vi "Actor Core.vi"(8 "error in":errorcluster, 11 "FlexUIActorTemplate in":refnum<class "FlexUIActorTemplate.lvclass">) -> (0 "error out":errorcluster, 3 "Actor out":refnum<class "Actor.lvclass">)   [LabVIEW 2016, in "FlexUIActorTemplate.lvlib" / "FlexUIActorTemplate.lvclass"]
doc: "(<B>Filename</B>: Actor Framework.lvlib:Actor.lvclass:Actor Core.vi)\n\nReceives messages to the actor, reacts to them, and initiates any error handling that may shut the actor down.\n\nDescendant classes may override this VI to append parallel tasks for the actor to complete while it handles messages. Overrides use the Call Parent Method node."
uses:
  FlexUIActorTemplate.lvclass
  <vilib>/ActorFramework/Actor/Actor.lvclass
  Flex UI Dialog (Actor) Messages/Publish UI Closed Msg/Publish UI Closed Msg.lvclass
  <vilib>/ActorFramework/Stop Msg/Stop Msg.lvclass
  Flex UI Dialog (Actor)/Flex Dialog (Actor).lvclass
  E:/LabVIEW/VI Packages/Flex UI (Actor)/Flex UI Dialog (Actor)/Flex Dialog (Actor).lvclass
  E:/LabVIEW/VI Packages/Flex UI (Actor)/Flex UI (Actor)/Flex UI (Actor).lvclass
  C:/Program Files (x86)/National Instruments/LabVIEW 2016/vi.lib/East West Architects/Parent Actor Template/_Parent Actor Template.lvclass
  C:/Program Files (x86)/National Instruments/LabVIEW 2016/vi.lib/ActorFramework/Actor/Actor.lvclass
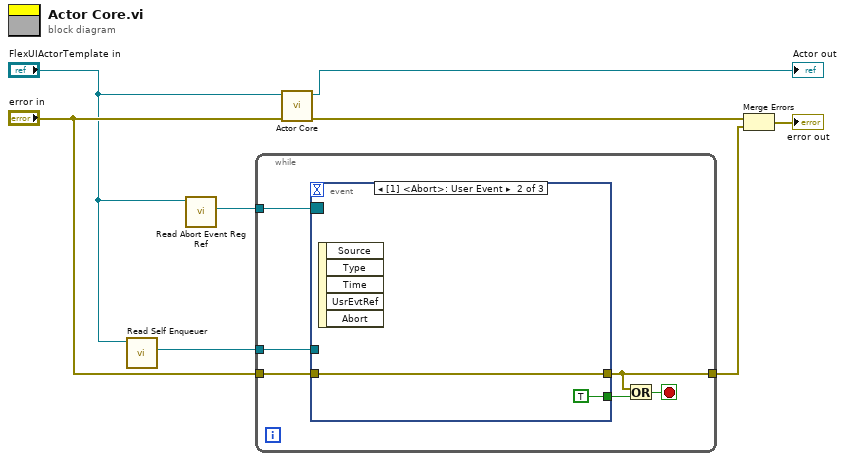
[diagram p0: block diagram]
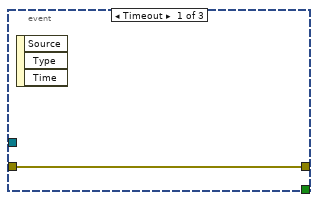
[diagram p2: hidden frame]
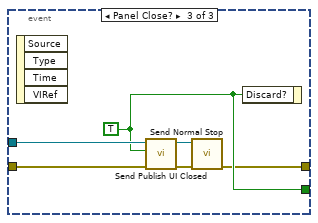
[diagram p3: hidden frame]
diagram:
  n1 = call <vilib>:"Read Self Enqueuer.vi"("Actor"="FlexUIActorTemplate in") -> ("Self Enqueuer"=w5:refnum<class "Message Enqueuer.lvclass">)  [unwired: 10 in]
  n2 = call-dynamic "Read Abort Event Reg Ref.vi"("Flex  Dialog (Actor) in"="FlexUIActorTemplate in") -> ("Abort Event Reg Ref"=w2:refnum<event-registration>)  [unwired: 9 in, 1 out]
  n3 = while {
    tunnel: "error in" -> [w14]
    tunnel: [w13] -> w3
    tunnel: w5 -> [w12]
    tunnel: w2 -> [w9]
    stop <- w10 stop-if-true
    n4 = event shown="[1] <Abort>: User Event" {
      selector: w9 -> [_ _ _]
      dyn-events: _ -> [_ _ _]
      timeout: _ -> [_ _ _]
      tunnel: w14 -> [w15 w16 w23]
      tunnel: [w15 w16 w19] -> w13
      tunnel: w12 -> [_ _ w21]
      tunnel: [_ TRUE w20] -> w11
      event Timeout {
        n5 = event-data() -> ()  [unwired: 1 in, 3 out]
      }
      event User Event {
        n6 = event-data() -> ()  [unwired: 1 in, 5 out]
      }
      event Panel Close? {
        w20 = TRUE ("Closed")
        n7 = event-data() -> ()  [unwired: 1 in, 4 out]
        n8 = call "Send Publish UI Closed.vi"("error in (no error)"=w23, "Closed"=w20, "Message Enqueuer in"=w21) -> ("error out"=w22:errorcluster, "Message Enqueuer out"=w18:refnum<class "Message Enqueuer.lvclass">)  [unwired: 7 in]
        n9 = call <vilib>:"Send Normal Stop.vi"("error in (no error)"=w22, "Message Enqueuer"=w18) -> ("error out"=w19:errorcluster)  [unwired: 9 in]
        n10 = event-data("Discard?"=w20) -> ()  [unwired: 1 in, 1 out]
      }
    }
    n11 = Or(x=w13, y=w11) -> (x .or. y?=w10:bool)
  }
  n12 = call-parent "Actor Core.vi"("error in"="error in", "Flex UI (Actor) in"="FlexUIActorTemplate in") -> ("error out"=w8:errorcluster, "Actor out"=→"Actor out":refnum<class "Actor.lvclass">)  [unwired: 8 in]
  n13 = Merge Errors(w8, w3) -> (→"error out":errorcluster)
